vi "GetHighPrioritySensors.vi"() -> ()   [LabVIEW 2020]
doc: "All high priority sensor reads and safety interlock calculations should be placed in this VI."
uses:
  GlobalMiscellaneous.vi
  GlobalArm.vi
  GlobalDriverStationData.vi
  GlobalDrivebase.vi
  GRNF_POT.vi
  GlobalGripper.vi
  GRNF_GenericSolenoid.vi
  <vilib>/Rock Robotics/WPI/Solenoid/Deprecated/WPI_SolenoidGetBool.vi
  GlobalHopper.vi
  GRNF_ColorSensor.vi
panel:
  in  "Gripper Game Piece Detection Time (ms)":u32=200
  out "Wrist":dbl
  out "Elbow":dbl
  out "Shoulder":dbl
  out "End Effector Position (in)":dbl[](array[numeric]) format="%#.1f"
  in  "Hopper Game Piece Detection Time (ms)":u32=50
  in  "Game Piece Proximity Threshold":u16=325
  out "Raw Color":u32(colorbox)
  out "Color Sensor Proximity":u16
  # "X"
  # "Y"
  # "Z"
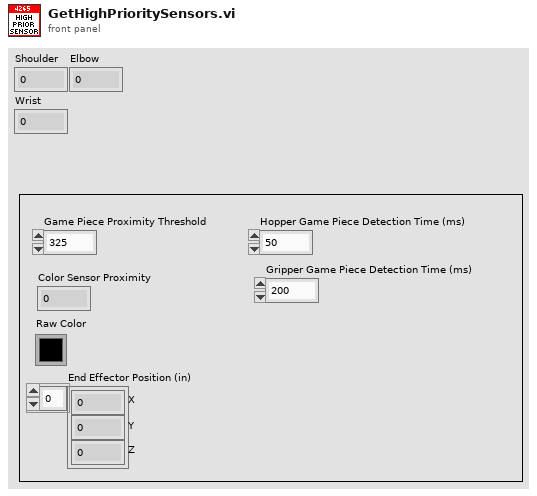
[diagram p1: front panel]
types:
  T1 = enum16{"Low Gear", "High Gear", "Transiting", "Unknown", "Force Low Gear"}
  T2 = typedef "Color Sensor V3 DevRef.ctl" = cluster{"I2CDevRef":T3}
  T3 = typedef "WPI_I2CDevRef.ctl" = cluster{"DevStatus":errorcluster, "Device Address":u8, "Handle":i32, "I2C Bus":T4}
  T4 = typedef "i2c_bus.ctl" = enum16{"I2C On-Board", "I2C MXP", "Invalid"}
  T5 = typedef "WPI_PotentiometerDevRef.ctl" = cluster{"DevStatus":errorcluster, "Analog Channel":T6, "Invert Output":bool}
  T6 = typedef "FPGA_AIChannel.ctl" = enum8{"AI 0", "AI 1", "AI 2", "AI 3", "AI MXP 0", "AI MXP 1", "AI MXP 2", "AI MXP 3", "Invalid"}
  T7 = typedef "WPI_DigitalInputDevRef.ctl" = cluster{"DevStatus":errorcluster, "DIO Channel":T8}
  T8 = typedef "FPGA_DIOChannel.ctl" = enum8{"DIO 0", "DIO 1", "DIO 2", "DIO 3", "DIO 4", "DIO 5", "DIO 6", "DIO 7", "DIO 8", "DIO 9", "DIO MXP 0", "DIO MXP 1", "DIO MXP 2", "DIO MXP 3", "DIO MXP 4", "DIO MXP 5", "DIO MXP 6", "DIO MXP 7", "DIO MXP 8", "DIO MXP 9", "DIO MXP 10", "DIO MXP 11", "DIO MXP 12", "DIO MXP 13", "DIO MXP 14", "DIO MXP 15", "SPI Port CS1", "SPI Port CS2", "SPI Port CS3", "SPI Port MISO", "SPI Port MOSI", "Invalid"}
  T9 = typedef "WPI_SolenoidDevRef.ctl" = cluster{"DevStatus":errorcluster, "Pneumatics Control Module":u8, "Forward Solenoid Channel":T10, "Reverse Solenoid Channel":T10}
  T10 = typedef "WPI_SolenoidChannel.ctl" = enum8{"Solenoid 0", "Solenoid 1", "Solenoid 2", "Solenoid 3", "Solenoid 4", "Solenoid 5", "Solenoid 6", "Solenoid 7", "Solenoid 8", "Solenoid 9", "Solenoid 10", "Solenoid 11", "Solenoid 12", "Solenoid 13", "Solenoid 14", "Solenoid 15", "Invalid"}
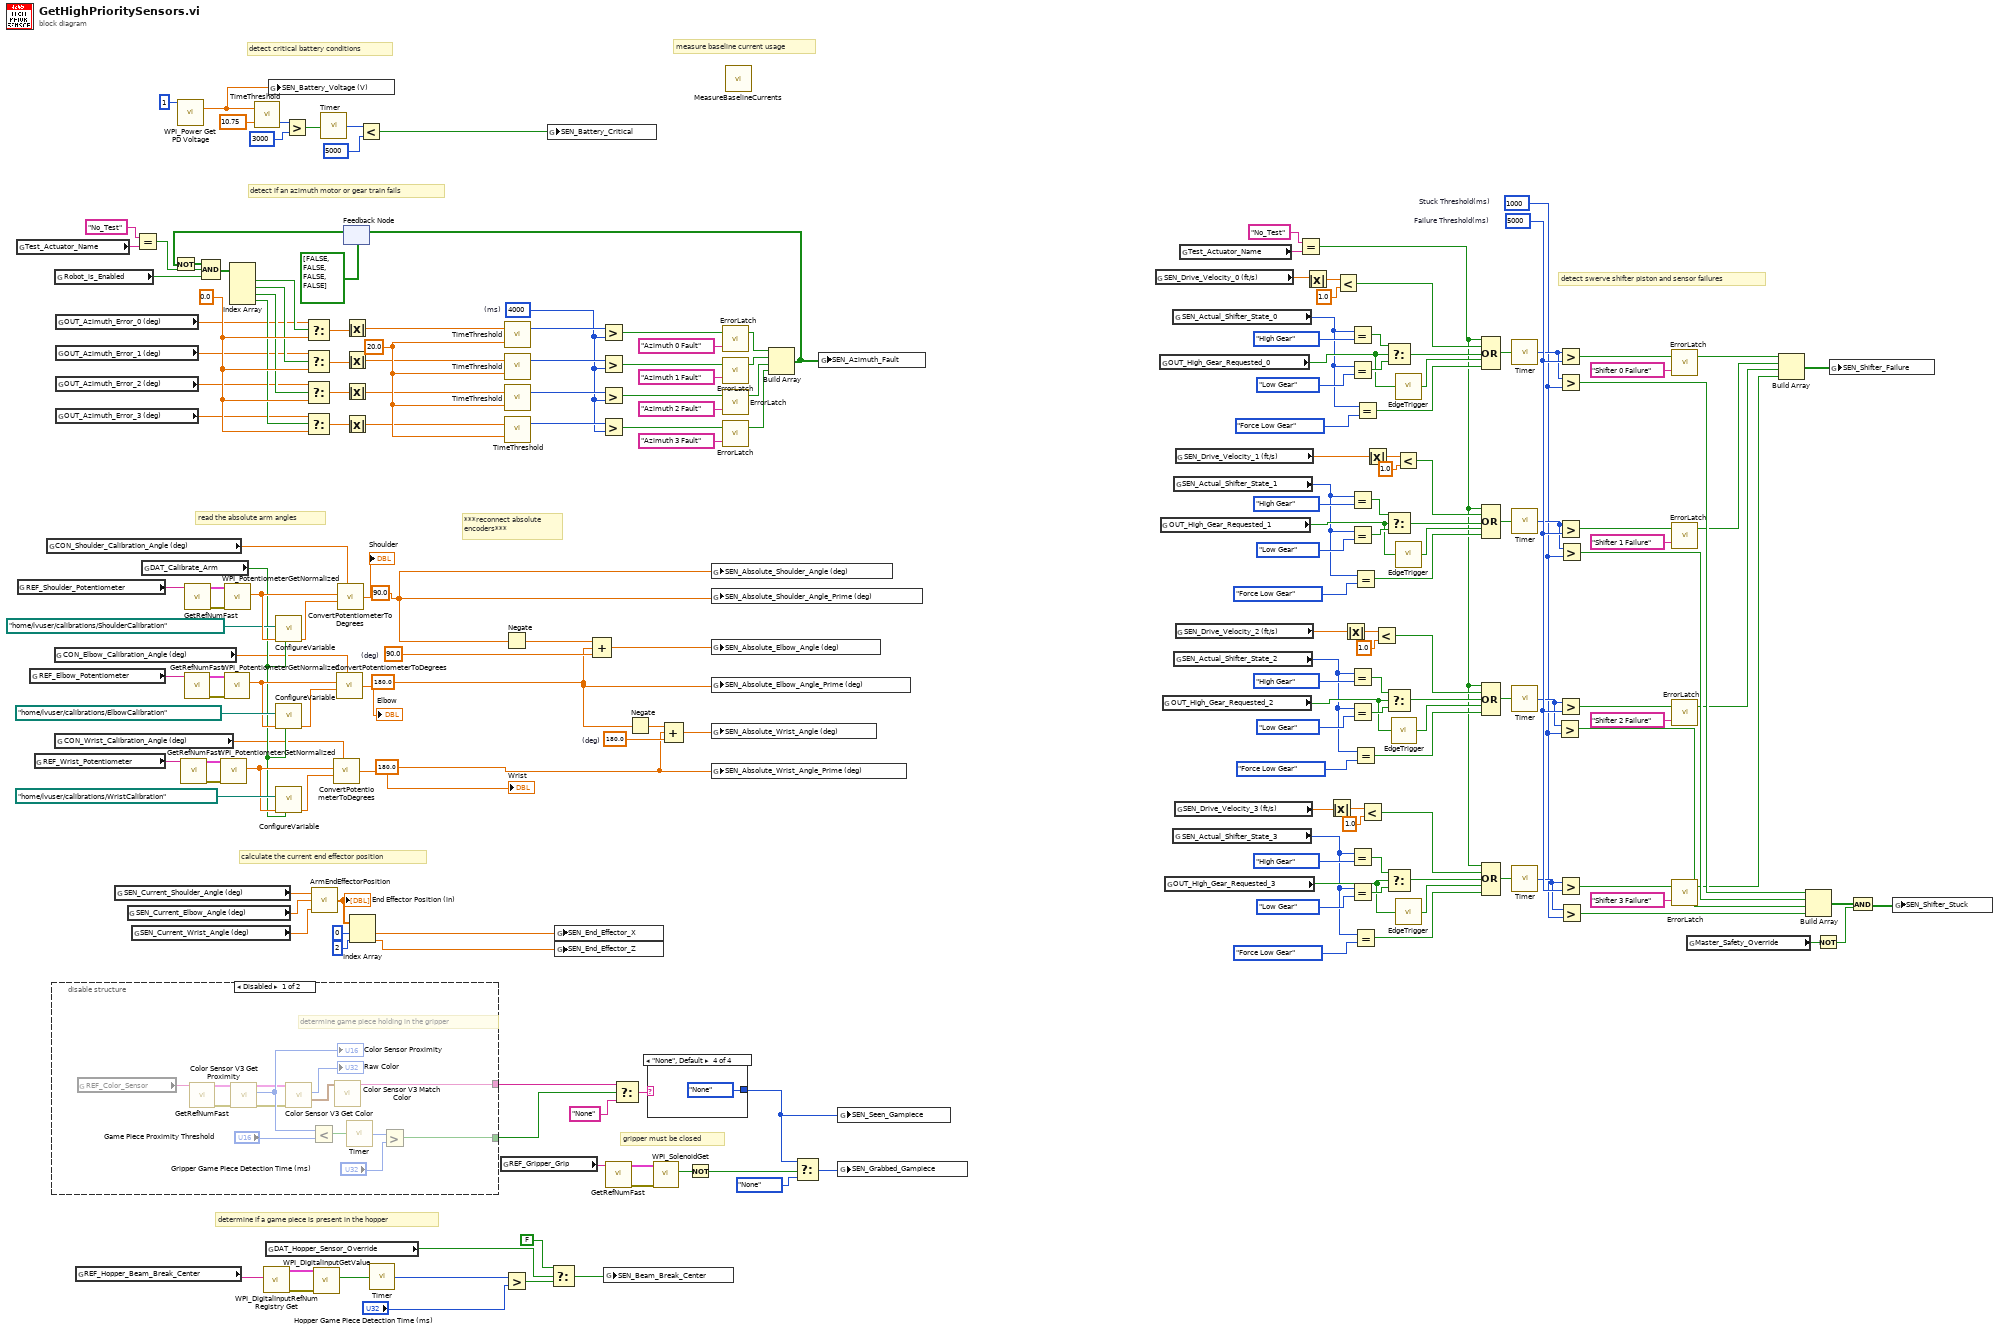
[diagram p0: block diagram]
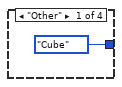
[diagram p3: hidden frame]
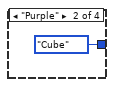
[diagram p4: hidden frame]
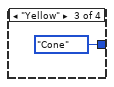
[diagram p5: hidden frame]
diagram:
  w12 = 180.0
  w13 = 180.0
  w14 = 90.0
  w28 = 180.0  # (deg)
  w30 = 90.0  # (deg)
  w150 = u32 1000  # Stuck Threshold(ms)
  w167 = u32 5000  # Failure Threshold(ms)
  w116 = 0.0
  w200 = u32 4000  # (ms)
  w199 = 20.0 ("Threshold")
  # "calculate the current end effector position"
  # "***reconnect absolute\nencoders***"
  # "determine if a game piece is present in the hopper"
  # "gripper must be closed"
  # "read the absolute arm angles"
  # "measure baseline current usage"
  # "detect critical battery conditions"
  # "detect swerve shifter piston and sensor failures"
  # "detect if an azimuth motor or gear train fails"
  n1 = global read "GlobalDriverStationData.vi" "Test_Actuator_Name"() -> (w74:string)
  n2 = global read "GlobalArm.vi" "REF_Shoulder_Potentiometer"() -> (w65:string)
  n3 = global read "GlobalArm.vi" "REF_Elbow_Potentiometer"() -> (w62:string)
  n4 = global read "GlobalArm.vi" "REF_Wrist_Potentiometer"() -> (w59:string)
  n5 = global read "GlobalArm.vi" "CON_Shoulder_Calibration_Angle (deg)"() -> (w45:dbl)
  n6 = disable-structure shown="Disabled" {
    disable-tunnel: [w221 _] -> w51
    disable-tunnel: [w208 _] -> w4
    frame Disabled {
      # "determine game piece holding in the gripper"
      n7 = global read "GlobalGripper.vi" "REF_Color_Sensor"() -> (w212:string)
      n8 = call-poly "GetRefNumFast.vi"("RefNum Name"=w212) -> ("Error"=w213:errorcluster, "Device Reference"=w214:T2)  [unwired: 5 in]
      n9 = call <vilib>:"Color Sensor V3 Get Proximity.vi"("error in (no error)"=w213, "ColorSensorDevRef"=w214) -> ("error out"=w215:errorcluster, "Proximity"=w219:u16, "ColorSensorDevRef out"=w216:T2)  [unwired: 7 in]
      "Color Sensor Proximity" <- w219
      n10 = call <vilib>:"Color Sensor V3 Get Color.vi"("error in (no error)"=w215, "ColorSensorDevRef"=w216) -> ("Normalized Color"=w220:cluster{"R":dbl, "G":dbl, "B":dbl}, "Color"=→"Raw Color":u32)  [unwired: 6 in, 2 out]
      n11 = Less?(x=w219, y="Game Piece Proximity Threshold") -> (x < y?=w210:bool)
      n12 = call <vilib>:"Color Sensor V3 Match Color.vi"("Measured Color"=w220) -> ("Matched Color Name"=w221:string)  [unwired: 8 in, 2 out]
      n13 = call "Timer.vi"("Reset Timer"=w210) -> ("Time (ms)"=w209:u32)
      n14 = Greater?(x=w209, y="Gripper Game Piece Detection Time (ms)") -> (0:w208:bool)
    }
    frame Enabled {
    }
  }
  n15 = global read "GlobalArm.vi" "CON_Elbow_Calibration_Angle (deg)"() -> (w44:dbl)
  n16 = global read "GlobalDriverStationData.vi" "Robot_is_Enabled"() -> (w68:bool)
  n17 = global read "GlobalArm.vi" "CON_Wrist_Calibration_Angle (deg)"() -> (w43:dbl)
  n18 = global read "GlobalDrivebase.vi" "OUT_Azimuth_Error_0 (deg)"() -> (w93:dbl)
  n19 = global read "GlobalDrivebase.vi" "OUT_Azimuth_Error_1 (deg)"() -> (w92:dbl)
  n20 = global read "GlobalDrivebase.vi" "OUT_Azimuth_Error_2 (deg)"() -> (w91:dbl)
  n21 = global read "GlobalDrivebase.vi" "OUT_Azimuth_Error_3 (deg)"() -> (w90:dbl)
  n22 = global read "GlobalHopper.vi" "REF_Hopper_Beam_Break_Center"() -> (w38:string)
  n23 = global read "GlobalArm.vi" "SEN_Current_Shoulder_Angle (deg)"() -> (w25:dbl)
  n24 = global read "GlobalArm.vi" "SEN_Current_Elbow_Angle (deg)"() -> (w24:dbl)
  n25 = global read "GlobalArm.vi" "SEN_Current_Wrist_Angle (deg)"() -> (w23:dbl)
  n26 = Equal?(x="No_Test", y=w74) -> (x = y?=w73:bool)
  n27 = global read "GlobalArm.vi" "DAT_Calibrate_Arm"() -> (w52:bool)
  n28 = call <vilib>:"WPI_Power Get PD Voltage.vi"("Power Distribution Panel (def)"=u8 1) -> ("voltage (V)"=w77:dbl)  [unwired: 13 in, 1 out]
  n29 = call-poly "GetRefNumFast.vi"("RefNum Name"=w59) -> ("Error"=w60:errorcluster, "Device Reference"=w61:T5)  [unwired: 5 in]
  n30 = call-poly "GetRefNumFast.vi"("RefNum Name"=w62) -> ("Error"=w63:errorcluster, "Device Reference"=w64:T5)  [unwired: 5 in]
  n31 = call-poly "GetRefNumFast.vi"("RefNum Name"=w65) -> ("Error"=w66:errorcluster, "Device Reference"=w67:T5)  [unwired: 5 in]
  n32 = call <vilib>:"WPI_PotentiometerGetNormalized.vi"("error in"=w60, "PotDevRef"=w61) -> ("Normalized Value"=w53:dbl)  [unwired: 7 in, 2 out]
  n33 = call <vilib>:"WPI_PotentiometerGetNormalized.vi"("error in"=w63, "PotDevRef"=w64) -> ("Normalized Value"=w55:dbl)  [unwired: 7 in, 2 out]
  n34 = call <vilib>:"WPI_PotentiometerGetNormalized.vi"("error in"=w66, "PotDevRef"=w67) -> ("Normalized Value"=w58:dbl)  [unwired: 7 in, 2 out]
  n35 = call "TimeThreshold.vi"("Threshold"=10.75, "Current Value"=w77) -> ("Time Below Threshold (ms)"=w206:u32)  [unwired: 1 out]
  n36 = call <vilib>:"WPI_DigitalInputRefNum Registry Get.vi"("refnum name"=w38) -> ("error out"=w36:errorcluster, "DigitalInputDevRef"=w37:T7)  [unwired: 9 in]
  n37 = global read "GlobalDrivebase.vi" "DAT_Hopper_Sensor_Override"() -> (w9:bool)
  n38 = global write "GlobalMiscellaneous.vi" "SEN_Battery_Voltage (V)"(w77) -> ()
  n39 = call "ConfigureVariable.vi"("Apply New Setpoint"=w52, "New Setpoint Value"=w58, "Setpoint Save Location"=path "/home/lvuser/calibrations/ShoulderCalibration") -> ("Selected Setpoint Value"=w48:dbl)  [unwired: 8 in]
  n40 = call "ConfigureVariable.vi"("Apply New Setpoint"=w52, "New Setpoint Value"=w55, "Setpoint Save Location"=path "/home/lvuser/calibrations/ElbowCalibration") -> ("Selected Setpoint Value"=w47:dbl)  [unwired: 8 in]
  n41 = call "ConfigureVariable.vi"("Apply New Setpoint"=w52, "New Setpoint Value"=w53, "Setpoint Save Location"=path "/home/lvuser/calibrations/WristCalibration") -> ("Selected Setpoint Value"=w46:dbl)  [unwired: 8 in]
  n42 = Greater?(x=w206, y=u32 3000) -> (0:w100:bool)
  n43 = call "ArmEndEffectorPosition.vi"("Wrist Angle (deg)"=w23, "Elbow Angle (deg)"=w24, "Shoulder Angle (deg)"=w25) -> ("Translation Vector (in)"=w22:dbl[])
  "End Effector Position (in)" <- w22
  n44 = call <vilib>:"WPI_DigitalInputGetValue.vi"("error in (no error)"=w36, "DigitalInputDevRef"=w37) -> ("Value"=w17:bool)  [unwired: 7 in, 2 out]
  n45 = call "Timer.vi"("Reset Timer"=w100) -> ("Time (ms)"=w99:u32)
  n46 = call "ConvertPotentiometerToDegrees.vi"("Calibration Angle (deg)"=w43, "Potentiometer Calibration Value [0-1]"=w46, "Raw Potentiometer Value [0,1]"=w53) -> ("Orientation (deg) [-180,+180]"=→"Wrist":dbl)  [unwired: 3 in]
  n47 = call "ConvertPotentiometerToDegrees.vi"("Calibration Angle (deg)"=w44, "Potentiometer Calibration Value [0-1]"=w47, "Raw Potentiometer Value [0,1]"=w55) -> ("Orientation (deg) [-180,+180]"=→"Elbow":dbl)  [unwired: 3 in]
  n48 = call "ConvertPotentiometerToDegrees.vi"("Calibration Angle (deg)"=w45, "Potentiometer Calibration Value [0-1]"=w48, "Raw Potentiometer Value [0,1]"=w58) -> ("Orientation (deg) [-180,+180]"=→"Shoulder":dbl)  [unwired: 3 in]
  n49 = feedback #1(bool[] [FALSE, FALSE, FALSE, FALSE]) -> (w115:bool[])
  n50 = Not(x=w115) -> (.not. x?=w76:bool[])
  n51 = Compound Arithmetic op=AND(w76, w73, w68) -> (w114:bool[])
  n52 = Index Array(array=w114) -> (element #1=w110:bool, element #2=w111:bool, element #3=w112:bool, element #4=w113:bool)  [unwired: 4 in]
  n53 = Select(t=w93, s=w110, f=w116) -> (s? t:f=w191:dbl)
  n54 = Select(t=w92, s=w111, f=w116) -> (s? t:f=w190:dbl)
  n55 = Select(t=w91, s=w112, f=w116) -> (s? t:f=w189:dbl)
  n56 = Select(t=w90, s=w113, f=w116) -> (s? t:f=w188:dbl)
  n57 = Absolute Value(x=w191) -> (abs(x)=w198:dbl)
  n58 = Absolute Value(x=w190) -> (abs(x)=w197:dbl)
  n59 = Absolute Value(x=w189) -> (abs(x)=w196:dbl)
  n60 = Absolute Value(x=w188) -> (abs(x)=w195:dbl)
  n61 = Index Array(array=w22, index #1=0 ("index"), index #2=2 ("index")) -> (element #1=w19:dbl, element #2=w18:dbl)
  n62 = Less?(x=w99, y=u32 5000) -> (x < y?=w78:bool)
  n63 = call "Timer.vi"("Reset Timer"=w17) -> ("Time (ms)"=w35:u32)
  n64 = global read "GlobalGripper.vi" "REF_Gripper_Grip"() -> (w41:string)
  n65 = Negate(x=w14) -> (-x=w31:dbl)
  n66 = Greater?(x=w35, y="Hopper Game Piece Detection Time (ms)") -> (0:w11:bool)
  n67 = call "TimeThreshold.vi"("Threshold"=w199, "Current Value"=w198) -> ("Time Above Threshold (ms)"=w204:u32)  [unwired: 1 out]
  n68 = call "TimeThreshold.vi"("Threshold"=w199, "Current Value"=w197) -> ("Time Above Threshold (ms)"=w203:u32)  [unwired: 1 out]
  n69 = call "TimeThreshold.vi"("Threshold"=w199, "Current Value"=w196) -> ("Time Above Threshold (ms)"=w202:u32)  [unwired: 1 out]
  n70 = call "TimeThreshold.vi"("Threshold"=w199, "Current Value"=w195) -> ("Time Above Threshold (ms)"=w201:u32)  [unwired: 1 out]
  n71 = global write "GlobalMiscellaneous.vi" "SEN_Battery_Critical"(w78) -> ()
  n72 = Select(t=FALSE, s=w9, f=w11) -> (s? t:f=w10:bool)
  n73 = global write "GlobalArm.vi" "SEN_End_Effector_X"(w19) -> ()
  n74 = global write "GlobalArm.vi" "SEN_End_Effector_Z"(w18) -> ()
  n75 = Compound Arithmetic op=unknown(w31, w13, w30) -> (w26:dbl)
  n76 = Greater?(x=w204, y=w200) -> (0:w194:bool)
  n77 = Greater?(x=w203, y=w200) -> (0:w193:bool)
  n78 = Greater?(x=w202, y=w200) -> (0:w118:bool)
  n79 = Greater?(x=w201, y=w200) -> (0:w192:bool)
  n80 = global write "GlobalHopper.vi" "SEN_Beam_Break_Center"(w10) -> ()
  n81 = call-poly "GetRefNumFast.vi"("RefNum Name"=w41) -> ("Error"=w39:errorcluster, "Device Reference"=w40:T9)  [unwired: 5 in]
  n82 = Select(t=w51, s=w4, f="None") -> (s? t:f=w49:string)
  n83 = Negate(x=w13) -> (-x=w29:dbl)
  n84 = case shown="\"None\", Default" w49 {
    tunnel: [enum16{"None", "Cube", "Cone"}."Cube" ("SEN_Piece_Held") enum16{"None", "Cube", "Cone"}."Cube" ("SEN_Piece_Held") enum16{"None", "Cube", "Cone"}."Cone" ("SEN_Piece_Held") enum16{"None", "Cube", "Cone"}."None" ("SEN_Piece_Held")] -> w16
    frame "Other" {
    }
    frame "Purple" {
    }
    frame "Yellow" {
    }
    frame "None", Default {
    }
  }
  n85 = call-poly <vilib>:"WPI_SolenoidGet.vi"("error in (no error)"=w39, "SolenoidDevRef"=w40) -> ("Value"=w33:bool)  [unwired: 7 in, 2 out]
  n86 = Compound Arithmetic op=unknown(w29, w12, w28) -> (w27:dbl)
  n87 = Not(x=w33) -> (.not. x?=w32:bool)
  n88 = global write "GlobalArm.vi" "SEN_Absolute_Shoulder_Angle (deg)"(w14) -> ()
  n89 = global write "GlobalArm.vi" "SEN_Absolute_Shoulder_Angle_Prime (deg)"(w14) -> ()
  n90 = global write "GlobalArm.vi" "SEN_Absolute_Elbow_Angle (deg)"(w26) -> ()
  n91 = global write "GlobalArm.vi" "SEN_Absolute_Elbow_Angle_Prime (deg)"(w13) -> ()
  n92 = global write "GlobalArm.vi" "SEN_Absolute_Wrist_Angle (deg)"(w27) -> ()
  n93 = global write "GlobalArm.vi" "SEN_Absolute_Wrist_Angle_Prime (deg)"(w12) -> ()
  n94 = call "ErrorLatch.vi"("Error Message"="Azimuth 0 Fault", "Trigger"=w194) -> ("Latched"=w72:bool)  [unwired: 1 in]
  n95 = call "ErrorLatch.vi"("Error Message"="Azimuth 1 Fault", "Trigger"=w193) -> ("Latched"=w71:bool)  [unwired: 1 in]
  n96 = call "ErrorLatch.vi"("Error Message"="Azimuth 2 Fault", "Trigger"=w118) -> ("Latched"=w70:bool)  [unwired: 1 in]
  n97 = call "ErrorLatch.vi"("Error Message"="Azimuth 3 Fault", "Trigger"=w192) -> ("Latched"=w69:bool)  [unwired: 1 in]
  n98 = call "MeasureBaselineCurrents.vi"() -> ()  [unwired: 12 in]
  n99 = Build Array(w72, w71, w70, w69) -> (w89:bool[])
  n100 = feedback-in #1(w89) -> ()
  n101 = Select(t=w16, s=w32, f=enum16{"None", "Cube", "Cone"}."None") -> (s? t:f=w15:enum16{"None", "Cube", "Cone"})
  n102 = global write "GlobalDrivebase.vi" "SEN_Azimuth_Fault"(w89) -> ()
  n103 = global write "GlobalGripper.vi" "SEN_Seen_Gampiece"(w16) -> ()
  n104 = global write "GlobalGripper.vi" "SEN_Grabbed_Gampiece"(w15) -> ()
  n105 = global read "GlobalDrivebase.vi" "SEN_Drive_Velocity_0 (ft/s)"() -> (w88:dbl)
  n106 = global read "GlobalDrivebase.vi" "OUT_High_Gear_Requested_0"() -> (w97:bool)
  n107 = global read "GlobalDrivebase.vi" "OUT_High_Gear_Requested_1"() -> (w96:bool)
  n108 = global read "GlobalDrivebase.vi" "OUT_High_Gear_Requested_2"() -> (w95:bool)
  n109 = global read "GlobalDrivebase.vi" "OUT_High_Gear_Requested_3"() -> (w94:bool)
  n110 = global read "GlobalDrivebase.vi" "SEN_Actual_Shifter_State_0"() -> (w87:T1)
  n111 = global read "GlobalDrivebase.vi" "SEN_Actual_Shifter_State_3"() -> (w82:T1)
  n112 = global read "GlobalDrivebase.vi" "SEN_Actual_Shifter_State_1"() -> (w85:T1)
  n113 = global read "GlobalDrivebase.vi" "SEN_Actual_Shifter_State_2"() -> (w83:T1)
  n114 = global read "GlobalDrivebase.vi" "SEN_Drive_Velocity_3 (ft/s)"() -> (w81:dbl)
  n115 = global read "GlobalDrivebase.vi" "SEN_Drive_Velocity_1 (ft/s)"() -> (w86:dbl)
  n116 = global read "GlobalDrivebase.vi" "SEN_Drive_Velocity_2 (ft/s)"() -> (w84:dbl)
  n117 = global read "GlobalDriverStationData.vi" "Test_Actuator_Name"() -> (w2:string)
  n118 = Equal?(x="No_Test", y=w2) -> (x = y?=w1:bool)
  n119 = Absolute Value(x=w88) -> (abs(x)=w146:dbl)
  n120 = Absolute Value(x=w81) -> (abs(x)=w137:dbl)
  n121 = Less?(x=w146, y=1.0) -> (x < y?=w144:bool)
  n122 = Absolute Value(x=w84) -> (abs(x)=w140:dbl)
  n123 = Equal?(x=w87, y=T1."High Gear") -> (x = y?=w186:bool)
  n124 = Equal?(x=w87, y=T1."Low Gear") -> (x = y?=w184:bool)
  n125 = Equal?(x=w85, y=T1."High Gear") -> (x = y?=w181:bool)
  n126 = Equal?(x=w85, y=T1."Low Gear") -> (x = y?=w179:bool)
  n127 = Equal?(x=w83, y=T1."High Gear") -> (x = y?=w176:bool)
  n128 = Equal?(x=w83, y=T1."Low Gear") -> (x = y?=w174:bool)
  n129 = Equal?(x=w82, y=T1."High Gear") -> (x = y?=w171:bool)
  n130 = Equal?(x=w82, y=T1."Low Gear") -> (x = y?=w169:bool)
  n131 = Equal?(x=w85, y=T1."Force Low Gear") -> (x = y?=w129:bool)
  n132 = Equal?(x=w83, y=T1."Force Low Gear") -> (x = y?=w131:bool)
  n133 = Equal?(x=w82, y=T1."Force Low Gear") -> (x = y?=w133:bool)
  n134 = Equal?(x=w87, y=T1."Force Low Gear") -> (x = y?=w127:bool)
  n135 = Less?(x=w137, y=1.0) -> (x < y?=w135:bool)
  n136 = Absolute Value(x=w86) -> (abs(x)=w143:dbl)
  n137 = Less?(x=w140, y=1.0) -> (x < y?=w138:bool)
  n138 = Select(t=w186, s=w97, f=w184) -> (s? t:f=w165:bool)
  n139 = Select(t=w181, s=w96, f=w179) -> (s? t:f=w162:bool)
  n140 = Select(t=w176, s=w95, f=w174) -> (s? t:f=w160:bool)
  n141 = Select(t=w171, s=w94, f=w169) -> (s? t:f=w157:bool)
  n142 = call "EdgeTrigger.vi"("Input Signal"=w95) -> ("All Edge Trigger"=w159:bool)  [unwired: 2 out]
  n143 = call "EdgeTrigger.vi"("Input Signal"=w97) -> ("All Edge Trigger"=w166:bool)  [unwired: 2 out]
  n144 = Less?(x=w143, y=1.0) -> (x < y?=w141:bool)
  n145 = call "EdgeTrigger.vi"("Input Signal"=w96) -> ("All Edge Trigger"=w163:bool)  [unwired: 2 out]
  n146 = call "EdgeTrigger.vi"("Input Signal"=w94) -> ("All Edge Trigger"=w155:bool)  [unwired: 2 out]
  n147 = Compound Arithmetic op=OR(w1, w144, w165, w166, w127) -> (w164:bool)
  n148 = Compound Arithmetic op=OR(w1, w141, w162, w163, w129) -> (w161:bool)
  n149 = Compound Arithmetic op=OR(w1, w138, w160, w159, w131) -> (w158:bool)
  n150 = Compound Arithmetic op=OR(w1, w135, w157, w155, w133) -> (w156:bool)
  n151 = call "Timer.vi"("Reset Timer"=w164) -> ("Time (ms)"=w154:u32)
  n152 = call "Timer.vi"("Reset Timer"=w161) -> ("Time (ms)"=w153:u32)
  n153 = call "Timer.vi"("Reset Timer"=w158) -> ("Time (ms)"=w152:u32)
  n154 = call "Timer.vi"("Reset Timer"=w156) -> ("Time (ms)"=w151:u32)
  n155 = Greater?(x=w152, y=w150) -> (0:w121:bool)
  n156 = Greater?(x=w154, y=w167) -> (0:w183:bool)
  n157 = Greater?(x=w154, y=w150) -> (0:w125:bool)
  n158 = Greater?(x=w153, y=w167) -> (0:w178:bool)
  n159 = Greater?(x=w152, y=w167) -> (0:w173:bool)
  n160 = Greater?(x=w151, y=w167) -> (0:w168:bool)
  n161 = Greater?(x=w153, y=w150) -> (0:w123:bool)
  n162 = Greater?(x=w151, y=w150) -> (0:w120:bool)
  n163 = call "ErrorLatch.vi"("Error Message"="Shifter 0 Failure", "Trigger"=w183) -> ("Latched"=w126:bool)  [unwired: 1 in]
  n164 = call "ErrorLatch.vi"("Error Message"="Shifter 1 Failure", "Trigger"=w178) -> ("Latched"=w124:bool)  [unwired: 1 in]
  n165 = call "ErrorLatch.vi"("Error Message"="Shifter 2 Failure", "Trigger"=w173) -> ("Latched"=w122:bool)  [unwired: 1 in]
  n166 = call "ErrorLatch.vi"("Error Message"="Shifter 3 Failure", "Trigger"=w168) -> ("Latched"=w119:bool)  [unwired: 1 in]
  n167 = global read "GlobalDriverStationData.vi" "Master_Safety_Override"() -> (w149:bool)
  n168 = Build Array(w126, w124, w122, w119) -> (w80:bool[])
  n169 = Build Array(w125, w123, w121, w120) -> (w148:bool[])
  n170 = Not(x=w149) -> (.not. x?=w147:bool)
  n171 = global write "GlobalDrivebase.vi" "SEN_Shifter_Failure"(w80) -> ()
  n172 = And(x=w148, y=w147) -> (x .and. y?=w79:bool[])
  n173 = global write "GlobalDrivebase.vi" "SEN_Shifter_Stuck"(w79) -> ()
